vi "LWXPS_GroupJogParametersSet.vi"(0 "XPS Reference IN":refnum<k24>, 1 "Group Name":string, 2 "Number of positioners":i32, 3 "Velocity IN":dbl[](array[numeric]), 4 "Acceleration IN":dbl[](array[numeric]), 5 "LabVIEW error IN":errorcluster) -> (14 "XPS Reference OUT":refnum<k24>, 15 "Returned error code":i32, 16 "Velocity OUT":dbl[](array[numeric]), 17 "Acceleration OUT":dbl[](array[numeric]), 18 "XPS Error String":string, 19 "LabVIEW error OUT":errorcluster)   [LabVIEW 2014]
uses:
  D:/XPSQ8_LabView_Library/Development/Source/Dll/Newport.XPS.CommandInterface.dll
  Dll/Newport.XPS.CommandInterface.dll
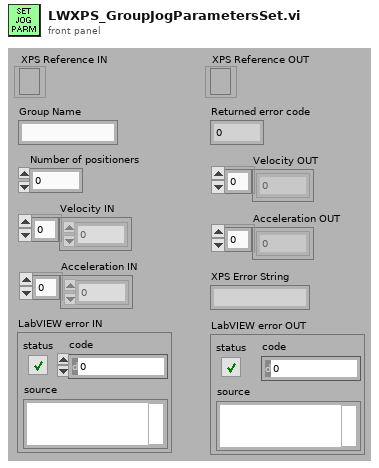
[diagram p1: front panel]
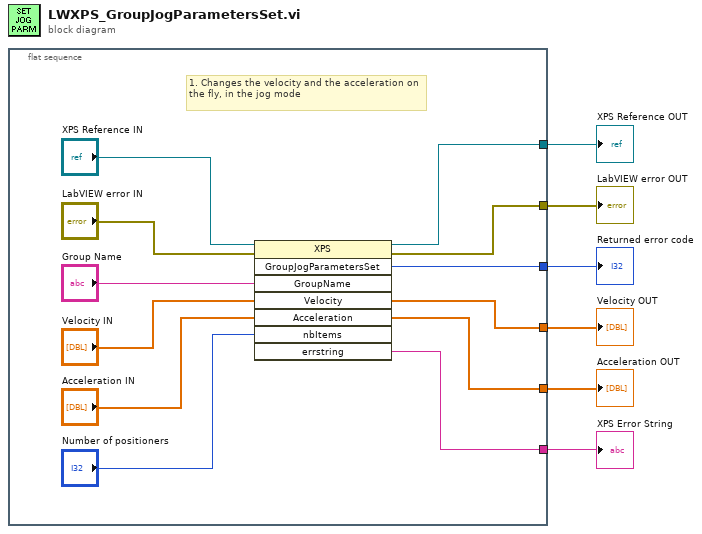
[diagram p0: block diagram]
diagram:
  n1 = flat-sequence {
    tunnel: [w10] -> w6
    tunnel: [w15] -> w5
    tunnel: [w17] -> w4
    tunnel: [w14] -> w2
    tunnel: [w9] -> w1
    tunnel: [w11] -> w3
    frame #0 {
      # "1. Changes the velocity and the acceleration on the fly, in the jog mode"
      n2 = invoke class="XPS" method="GroupJogParametersSet"(reference="XPS Reference IN", error in="LabVIEW error IN", "GroupName"="Group Name", "Velocity"="Velocity IN", "Acceleration"="Acceleration IN", "nbItems"="Number of positioners") -> (reference out=w10:refnum<k24>, error out=w15:errorcluster, "GroupJogParametersSet"=w17:i32, "Velocity"=w11:dbl[], "Acceleration"=w14:dbl[], "errstring"=w9:string)  [unwired: 2 in, 2 out]
    }
  }
  "XPS Reference OUT" <- w6
  "LabVIEW error OUT" <- w5
  "Returned error code" <- w4
  "XPS Error String" <- w1
  "Velocity OUT" <- w3
  "Acceleration OUT" <- w2
